vi "Upload File with Callback.vi"(7 "Remote Folder Path":string, 8 "error in (no error)":errorcluster, 9 "Connection Name":string, 10 "Local File Path":path, 11 "Remote File Name":string) -> (0 "error out":errorcluster, 3 "Return String":string)   [LabVIEW 2019, in "LabSFTP.lvlib"]
doc: "<License>This software is distributed under the BSD 3-Clause License. For the full license please see license.txt or visit www.labvolution.com/license</License>"
uses:
  LabSFTP.lvlib
  FGV State..enum.ctl
  C:/Users/1/Desktop/Pipeline leakage monitoring/V1.51-2020-8-10/References/LabSFTP.dll
  References/LabSFTP.dll
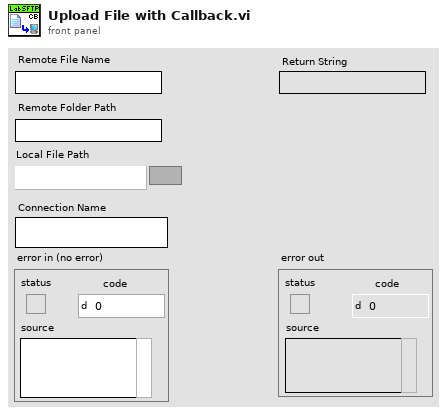
[diagram p1: front panel]
types:
  T1 = typedef "LabSFTP.lvlib/FGV State..enum.ctl" = enum16{"GET", "SET"}
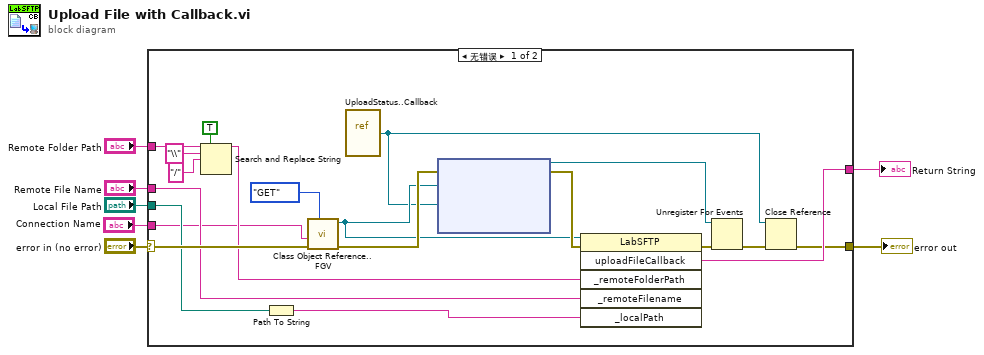
[diagram p0: block diagram]
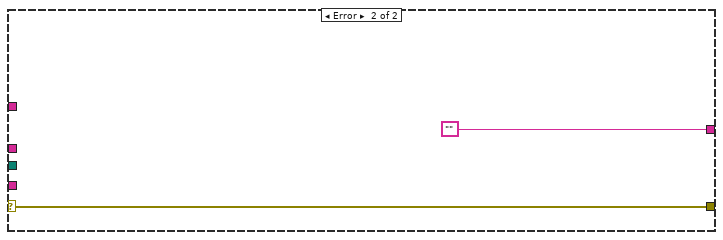
[diagram p2: hidden frame]
diagram:
  n1 = case shown="无错误" "error in (no error)" {
    selector: "error in (no error)" -> [w27 w29]
    tunnel: [w9 w29] -> w6
    tunnel: [w25 ""] -> w5
    tunnel: "Local File Path" -> [w24 _]
    tunnel: "Remote File Name" -> [w23 _]
    tunnel: "Remote Folder Path" -> [w18 _]
    tunnel: "Connection Name" -> [w16 _]
    frame No Error {
      n2 = Search and Replace String(replace all?=TRUE ("replace all? (F)"), input string=w18, search string="\\", replace string="/" ("replace string (\"\")")) -> (result string=w17:string)  [unwired: 4 in, 3 out]
      n3 = Path To String(path=w24) -> (string=w22:string)
      n4 = call "Class Object Reference..FGV.vi"("FGV State"=FGV_State..enum."GET", "error in (no error)"=w27, "Connection Name"=w16) -> ("error out"=w15:errorcluster, "LabSFTP ref out"=w13:refnum<k24>)  [unwired: 7 in]
      n5 = vi-ref "UploadStatus..Callback.vi"() -> (w8:refnum<vi>)
      n6 = node(w15, w13, w8) -> (w10:refnum<k27>, w14:errorcluster)  [unwired: 2 in]
      n7 = invoke class="LabSFTP" method="uploadFileCallback"(reference=w13, error in=w14, "_remoteFolderPath"=w17, "_remoteFilename"=w23, "_localPath"=w22) -> (error out=w12:errorcluster, "uploadFileCallback"=w25:string)  [unwired: 1 in, 4 out]
      n8 = Unregister For Events(event registration refnum=w10, error in=w12) -> (error out=w11:errorcluster)
      n9 = Close Reference(reference=w8, error in (no error)=w11) -> (error out=w9:errorcluster)
    }
    frame Error {
    }
  }
  "error out" <- w6
  "Return String" <- w5
